vi "DSP_SetFftLogeAmplMult.vi"(2 "error in (no error)":errorcluster, 3 "value":sgl, 4 "Board Handle":u64) -> (0 "error out":errorcluster, 1 "Board Handle Out":u64)   [LabVIEW 2009]
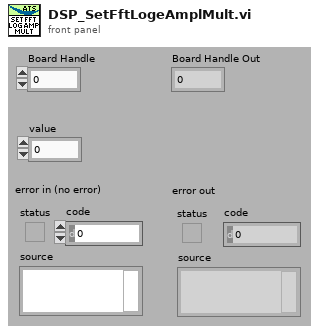
[diagram p1: front panel]
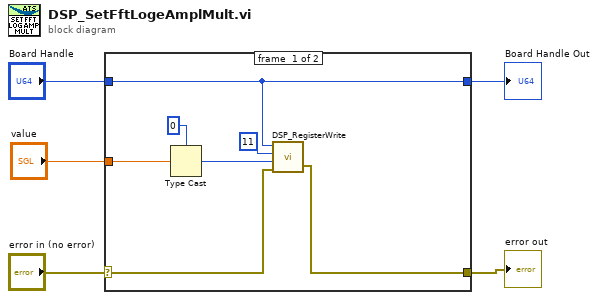
[diagram p0: block diagram]
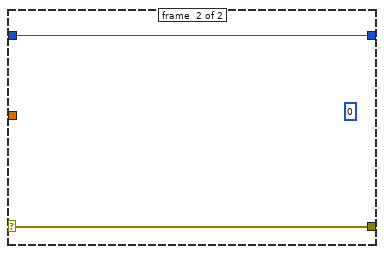
[diagram p2: hidden frame]
diagram:
  n1 = case shown="No Error" "error in (no error)" {
    selector: "error in (no error)" -> [w12 w14]
    tunnel: [w11 w14] -> w4
    tunnel: [w10 w13] -> w3
    tunnel: "Board Handle" -> [w10 w13]
    tunnel: "value" -> [w7 _]
    frame #0 {
      n2 = Type Cast(type=u32 0, x=w7) -> (*(type *) &x=w6:u32)
      n3 = call "DSP_RegisterWrite.vi"("error in (no error)"=w12, "Value"=w6, "Offset"=u32 11, "Board Handle"=w10) -> ("error out"=w11:errorcluster)  [unwired: 1 out]
    }
    frame #1 {
      (unwired) u32 0
    }
  }
  "Board Handle Out" <- w3
  "error out" <- w4
